vi "Sort Elcom Xp Array.vi"(1 "file path (dialog if empty)":path) -> (0 "subarray 3":string[][](array[string]))   [LabVIEW 2014]
uses:
  <vilib>/Utility/file.llb/Read From Spreadsheet File (string).vi
panel:
  out "Array":string[][](array[string])
  out "subarray 4":string[](array[string])
  out "size(s)":i32
  out "subarray 2":string[](array[string])
  out "element":i64
  out "appended array":i32[][](array[numeric])
  out "subarray":string[][](array[string])
  out "Sorted array":i64[][](array[numeric])
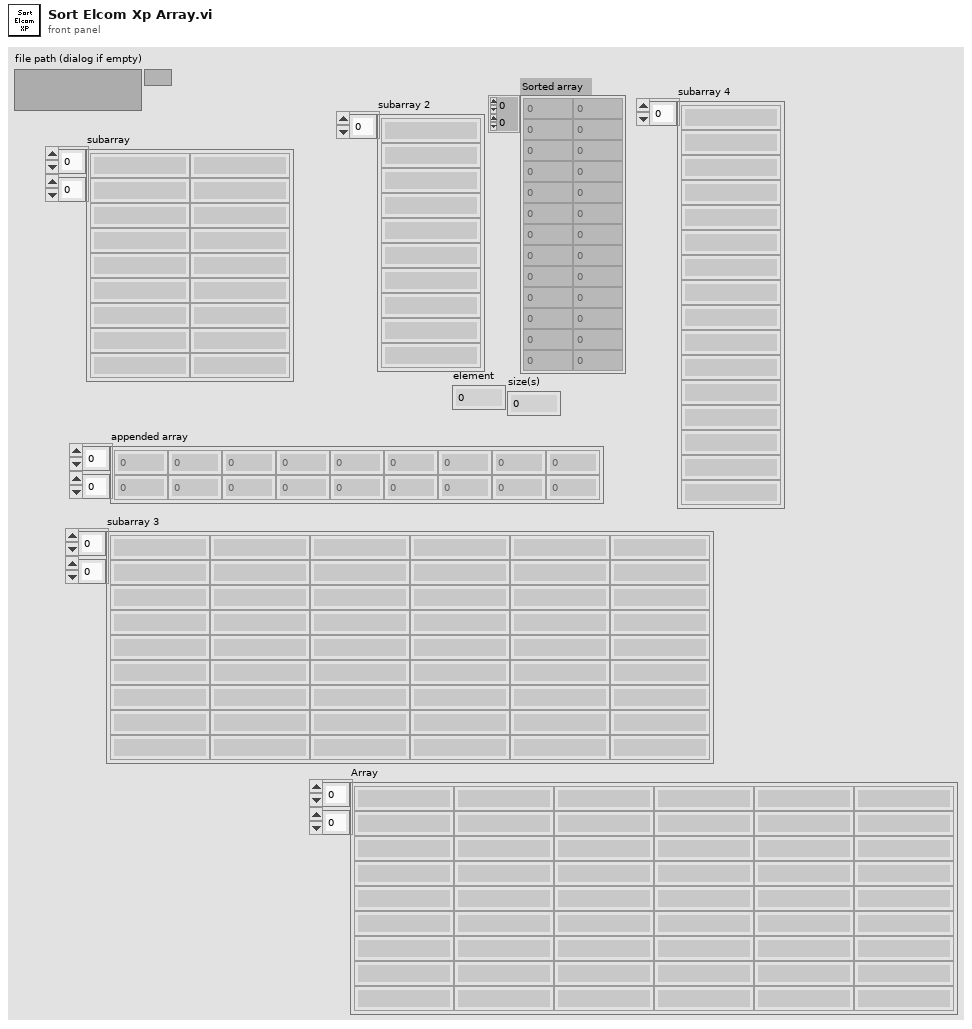
[diagram p1: front panel]
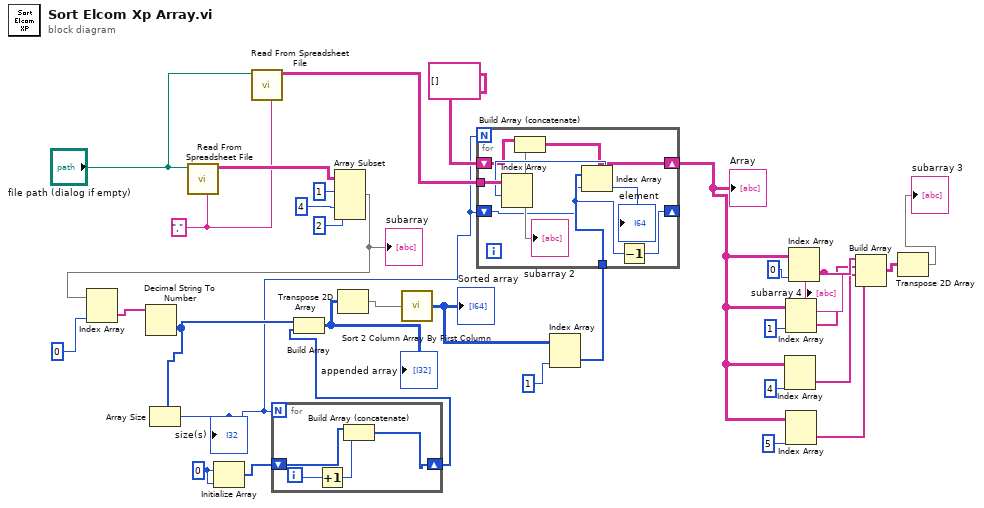
[diagram p0: block diagram]
diagram:
  w26 = 0 ("element")
  w14 = "," ("delimiter (\\t)")
  n1 = call-poly <vilib>:"Read From Spreadsheet File.vi"("delimiter (\\t)"=w14, "file path (dialog if empty)"="file path (dialog if empty)") -> ("all rows"=w32:string[][])  [unwired: 5 in, 4 out]
  n2 = Initialize Array(w26, w26) -> (w27:i32[])
  n3 = call-poly <vilib>:"Read From Spreadsheet File.vi"("delimiter (\\t)"=w14, "file path (dialog if empty)"="file path (dialog if empty)") -> ("all rows"=w16:string[][])  [unwired: 5 in, 4 out]
  n4 = Array Subset(array=w32, index (row)=1 ("index"), index (col)=4 ("index"), length (col)=2 ("length")) -> (w15:string[][])  [unwired: 1 in]
  "subarray" <- w15
  n5 = Index Array(array=w15, index (col)=0 ("index (row)")) -> (element=w25:string[])  [unwired: 1 in]
  n6 = Decimal String To Number(string=w25) -> (number=w24:i32[])  [unwired: 2 in, 1 out]
  n7 = Array Size(array=w24) -> (size(s)=w12:i32)
  "size(s)" <- w12
  n8 = for {
    N: w12 -> [_]
    shift-right: [w35] -> w23
    shift-left: w27 -> [w36]
    i -> [w34]
    n9 = Increment(x=w34) -> (x+1=w33:i32)
    n10 = Build Array (concatenate)(w36, w33) -> (w35:i32[])
  }
  n11 = Build Array(w24, w23) -> (w19:i32[][])
  "appended array" <- w19
  n12 = Transpose 2D Array(2D array=w19) -> (transposed array=w18:i32[][])
  n13 = call "Sort 2 Column Array By First Column.vi"("2D array to sort"=w18) -> ("Sorted array"=w22:i64[][])
  "Sorted array" <- w22
  n14 = Index Array(array=w22, index (col)=1 ("index (row)")) -> (element=w20:i64[])  [unwired: 1 in]
  n15 = for {
    N: w12 -> [_]
    tunnel: w20 -> [w43]
    tunnel: w16 -> [w44]
    shift-right: [w40] -> w9
    shift-left: string[][] [] ("Array") -> [w41]
    shift-right: [w37] -> _
    shift-left: w12 -> [w38]
    n16 = Index Array(array=w43, index=w38) -> (element=w42:i64)
    "element" <- w42
    n17 = Index Array(array=w44, index (row)=w42) -> (element=w39:string[])  [unwired: 1 in]
    "subarray 2" <- w39
    n18 = Build Array (concatenate)(w41, w39) -> (w40:string[][])
    n19 = Decrement(x=w38) -> (x-1=w37:i32)
  }
  "Array" <- w9
  n20 = Index Array(array=w9, index (col)=4 ("disabled index (col)")) -> (element=w4:string[])  [unwired: 1 in]
  n21 = Index Array(array=w9, index (col)=1 ("disabled index (col)")) -> (element=w5:string[])  [unwired: 1 in]
  n22 = Index Array(array=w9, index (col)=5 ("disabled index (col)")) -> (element=w3:string[])  [unwired: 1 in]
  n23 = Index Array(array=w9, index (col)=0 ("index (row)")) -> (element=w6:string[])  [unwired: 1 in]
  "subarray 4" <- w6
  n24 = Build Array(w6, w5, w4, w3) -> (w2:string[][])
  n25 = Transpose 2D Array(2D array=w2) -> (transposed array=→"subarray 3":string[][])
